vi "Compare Masters.vi"(8 "error in (no error)":errorcluster, 10 "All ECAT Masters":refnum<k21>[](array[refnum]), 11 "ECAT Master refs":T1[](array[typedef]) format="%.0x") -> (0 "error out":errorcluster, 3 "ECAT Masters":T2(array[cluster]) {"VS ref" format="%.0x"})   [LabVIEW 2020, in "SEECD Engine.lvlib"]
uses:
  SEECD Engine.lvlib
  <vilib>/NI VeriStand/Custom Device API/Custom Device Item Ref.ctl
  Shared/Globals/Property Strings.vi
  <vilib>/NI VeriStand/Custom Device API/Get Item Property (U32).vi
  Shared/Globals/Error Strings.vi
  <vilib>/NI VeriStand/Custom Device API/Custom Device API.lvlib
  Shared/SEECD Shared.lvlib
  <resource>/objmgr/IndComECAT.rc
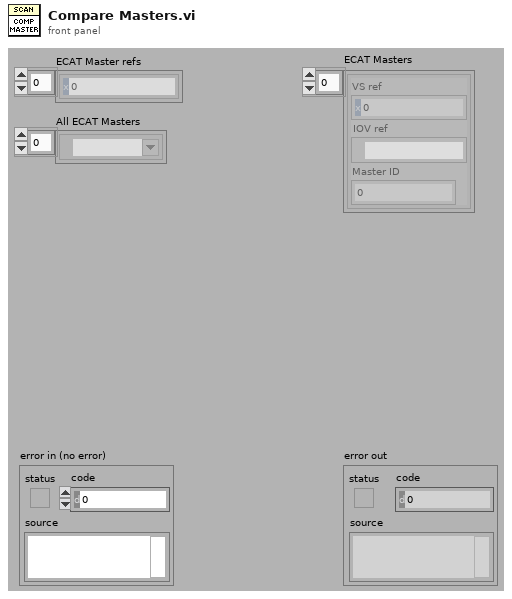
[diagram p1: front panel]
types:
  T1 = typedef "Custom Device API.lvlib/Custom Device Item Ref.ctl" = u64
  T2 = cluster{"VS ref":T1, "IOV ref":refnum<k21>, "Master ID":u32}[]
  T3 = cluster{"VS ref":T1, "IOV ref":refnum<k21>, "Master ID":u32}
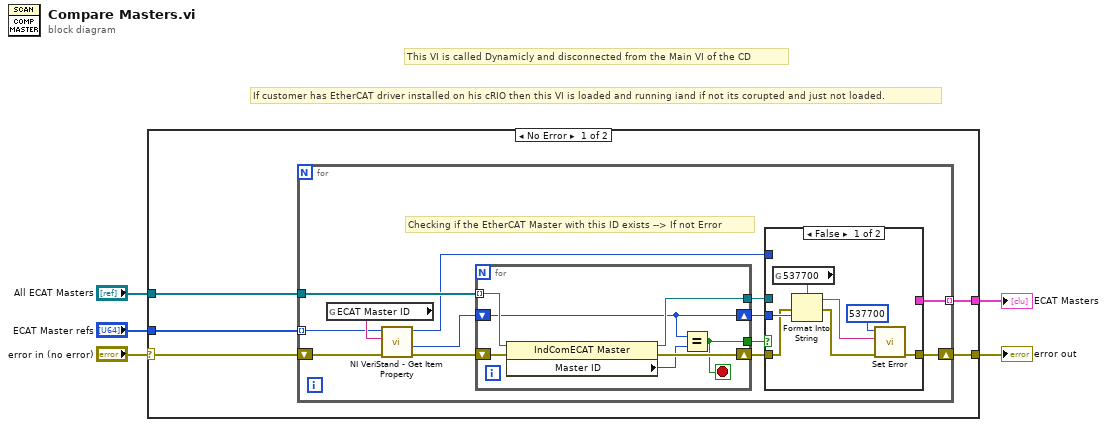
[diagram p0: block diagram]
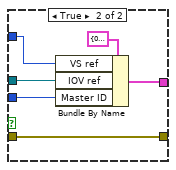
[diagram p2: hidden frame]
diagram:
  # "This VI is called Dynamicly and disconnected from the Main VI of the CD"
  # "If customer has EtherCAT driver installed on his cRIO then this VI is loaded and running iand if not its corupted and just not loaded."
  n1 = case shown="No Error" "error in (no error)" {
    selector: "error in (no error)" -> [w10 w44]
    tunnel: [w9 w44] -> w4
    tunnel: [w8 _] -> w3
    tunnel: "All ECAT Masters" -> [w7 _]
    tunnel: "ECAT Master refs" -> [w6 _]
    frame No Error {
      n2 = for {
        tunnel: w6 -> [w22] mode=indexing
        tunnel: w7 -> [w20]
        shift-right: [w16] -> w9
        shift-left: w10 -> [w21]
        tunnel: [w11] -> w8 mode=indexing
        # "Checking if the EtherCAT Master with this ID exists --> If not Error"
        n3 = global read "Property Strings.vi" "ECAT Master ID"() -> (w23:string)
        n4 = call-poly <vilib>:"NI VeriStand - Get Item Property.vi"("error in (no error)"=w21, "Property Name"=w23, "Item Ref in"=w22) -> ("error out"=w19:errorcluster, "Value"=w14:u32, "Item Ref out"=w15:T1)  [unwired: 5 in, 1 out]
        n5 = for {
          tunnel: w20 -> [w43] mode=indexing
          shift-right: [w41] -> w17
          shift-left: w19 -> [w42]
          tunnel: [w40] -> w18
          tunnel: [w39] -> w13
          shift-right: [w37] -> w12
          shift-left: w14 -> [w37]
          stop <- w40 stop-if-true
          n6 = property class="IndComECAT Master"(reference=w43, error in=w42) -> (reference out=w39:refnum<k21>, error out=w41:errorcluster, "Master ID"=w38:u32)
          n7 = Equal?(x=w37, y=w38) -> (x = y?=w40:bool)
        }
        n8 = case shown="False" w18 {
          tunnel: [w30 w31] -> w16
          tunnel: w17 -> [w27 w31]
          tunnel: w15 -> [_ w34]
          tunnel: w13 -> [_ w35]
          tunnel: w12 -> [w28 w32]
          tunnel: [_ w33] -> w11
          frame False {
            n9 = global read "Error Strings.vi" "537700"() -> (w29:string)
            n10 = Format Into String(format string=w29, error in=w27, w28) -> (resulting string=w25:string, error out=w26:errorcluster)  [unwired: 1 in]
            n11 = call "Set Error.vi"("error in (no error)"=w26, "Message"=w25, "Code"=537700) -> ("error out"=w30:errorcluster)  [unwired: 8 in]
          }
          frame True {
            n12 = Bundle By Name(cluster=T3 {"VS ref"=0, "IOV ref"="", "Master ID"=0} ("EtherCAT Master"), "VS ref"=w34, "IOV ref"=w35, "Master ID"=w32) -> (w33:T3)
          }
        }
      }
    }
    frame Error {
    }
  }
  "error out" <- w4
  "ECAT Masters" <- w3
